vi "write_command.vi"(8 "Arg":u8, 11 "Command":T1=enum."stop") -> ()   [LabVIEW 2011]
uses:
  Common/i2c_command.ctl
  <vilib>/rvi/DataTransferAndStorage/Container/Common/niFpgaContainerExecOnDevCompGetState.vi
  <vilib>/rvi/FIFO/Fifo_Resource/nirvififoEmulationSetSize.vi
  <vilib>/rvi/DataTransferAndStorage/Container/Common/niFpgaContainerGetUniqueNameForEmu.vi
  <vilib>/rvi/interface/RandomDataEmulation/nirviRandomDataFPGAFIFO.vi
  <vilib>/rvi/interface/RandomDataEmulation/niFpgaRandomDataHandleErrors.vi
  <vilib>/rvi/eio/common/nirviEmuReportErrorAndStop.vi
  <vilib>/rvi/DataTransferAndStorage/Container/XNode/niFpgaContainer.xnode
  <vilib>/rvi/FIFO/Fifo_Resource/niFpgaFifoEmulationRefIn.vi
panel:
  # "Write write a command with one arg byte to the bus controller."
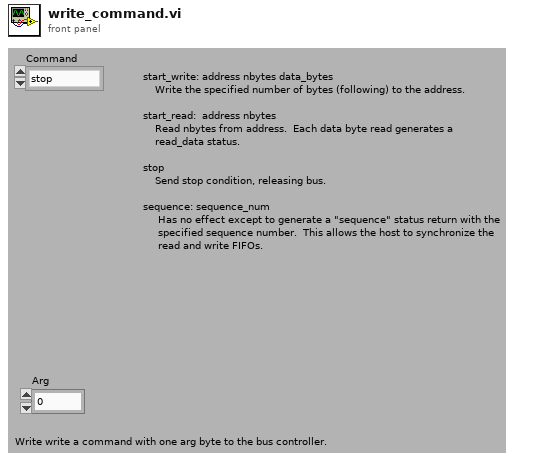
[diagram p1: front panel]
types:
  T1 = typedef "i2c_command.ctl" = enum8{"invalid", "start_write", "start_read", "stop", "sequence"}
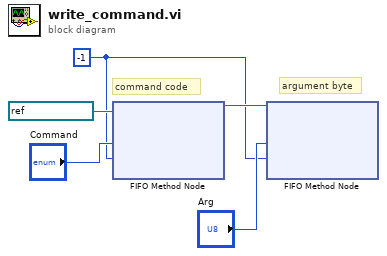
[diagram p0: block diagram]
diagram:
  w1 = -1 ("Timeout")
  # "argument byte"
  # "command code"
  n1 = xnode ("FIFO Method Node")("Element"="Command", "Timeout"=w1, "FIFO In"=refnum<k21> "Local write" ("FIFO")) -> ("FIFO Out"=w4:refnum<k21>)  [unwired: 1 out]
  n2 = xnode ("FIFO Method Node")("Element"="Arg", "Timeout"=w1, "FIFO In"=w4) -> ()  [unwired: 2 out]
